vi "getrfdivider.vi"(10 "Frequency (MHz)":dbl) -> (2 "RF Divider":i32)   [LabVIEW 2017]
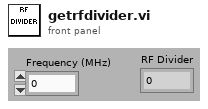
[diagram p1: front panel]
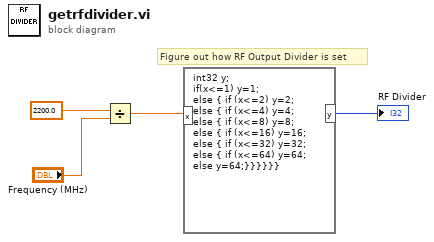
[diagram p0: block diagram]
diagram:
  # "Figure out how RF Output Divider is set"
  n1 = Divide(x=2200.0 ("y"), y="Frequency (MHz)") -> (x/y=w3:dbl)
  n2 = formula code="int32 y;\nif(x<=1) y=1;\nelse { if (x<=2) y=2;\nelse { if (x<=4) y=4;\nelse { if (x<=8) y=8;\nelse { if (x<=16) y=16;\nelse { if (x<=32) y=32;\nelse { if (x<=64) y=64;\nelse y=64;}}}}}}"("x"=w3) -> ("y"=→"RF Divider":i32)
